vi "Auto 11.vi"(8 "Error In":errorcluster, 11 "Forward?":bool) -> (0 "Error Out":errorcluster)   [LabVIEW 2014]
uses:
  <vilib>/Rock Robotics/Network Tables/SD Read Number.vi
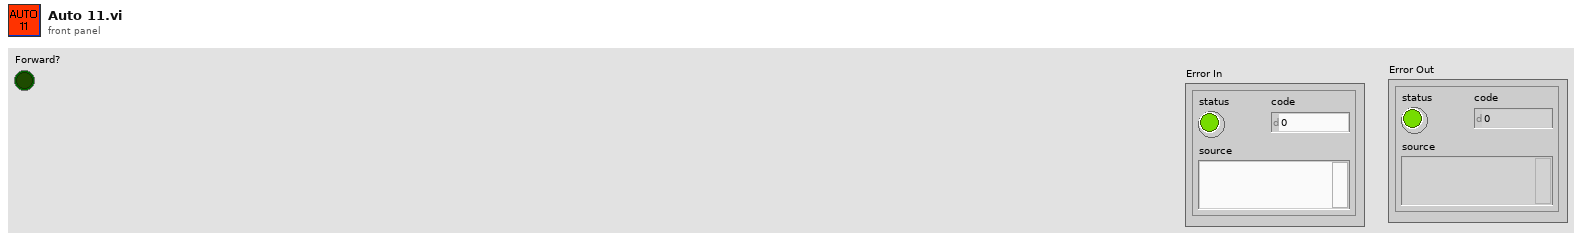
[diagram p1: front panel]
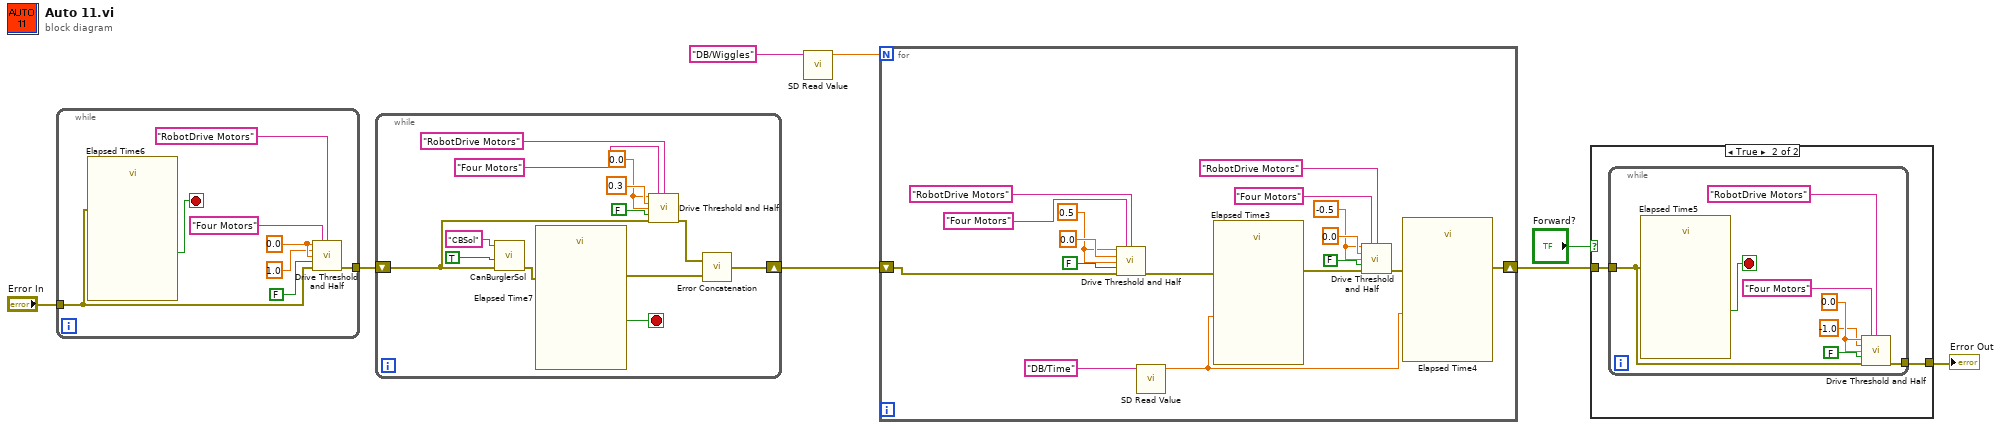
[diagram p0: block diagram]
diagram:
  n1 = while {
    tunnel: [w13] -> w3
    tunnel: "Error In" -> [w10]
    stop <- w11 stop-if-true
    w12 = 0.0 ("Arm Value")
    n2 = call "Elapsed Time6"("error in (no error)"=w10) -> ("Time has Elapsed"=w11:bool)  [unwired: 11 in, 7 out]
    n3 = call "Drive Threshold and Half.vi"("X In"=w12, "Drive refnum name"="Four Motors" ("refnum name"), "Send to DB Name"="RobotDrive Motors" ("Name"), "Y In"=1.0 ("X In"), "R In"=w12, "Speed Toggle"=FALSE ("Grabber Open/Close"), "Error In"=w10) -> ("Error Out"=w13:errorcluster)  [unwired: 8 in]
  }
  n4 = while {
    shift-right: [w17] -> w1
    shift-left: w3 -> [w20]
    stop <- w26 stop-if-true
    w24 = 0.0 ("Arm Value")
    n5 = call "CanBurglerSol.vi"("Error In"=w20, "Grabber Open/Close"=TRUE, "refnum name"="CBSol") -> ("Error Out"=w27:errorcluster)  [unwired: 8 in]
    n6 = call "Elapsed Time7"("error in (no error)"=w27) -> ("Time has Elapsed"=w26:bool, "error out"=w18:errorcluster)  [unwired: 11 in, 6 out]
    n7 = call "Drive Threshold and Half.vi"("X In"=w24, "Drive refnum name"="Four Motors" ("refnum name"), "Send to DB Name"="RobotDrive Motors" ("Name"), "Y In"=0.3 ("X In"), "R In"=w24, "Speed Toggle"=FALSE ("Grabber Open/Close"), "Error In"=w20) -> ("Error Out"=w19:errorcluster)  [unwired: 8 in]
    n8 = call "Error Concatenation.vi"("error in (no error) 2"=w18, "error in (no error)"=w19) -> ("error out"=w17:errorcluster)
  }
  n9 = call-poly <vilib>:"SD Read Value.vi"("Name"="DB/Wiggles") -> ("Numeric"=w4:dbl)  [unwired: 8 in, 2 out]
  n10 = for {
    N: w4 -> [_]
    shift-right: [w34] -> w7
    shift-left: w1 -> [w36]
    w31 = -0.5 ("Arm Value")
    w32 = 0.5 ("Arm Value")
    n11 = call "Drive Threshold and Half.vi"("X In"=w32, "Drive refnum name"="Four Motors" ("refnum name"), "Send to DB Name"="RobotDrive Motors" ("Name"), "Y In"=0.0 ("X In"), "R In"=w32, "Speed Toggle"=FALSE ("Grabber Open/Close"), "Error In"=w36) -> ("Error Out"=w42:errorcluster)  [unwired: 8 in]
    n12 = call-poly <vilib>:"SD Read Value.vi"("Name"="DB/Time") -> ("Numeric"=w30:dbl)  [unwired: 8 in, 2 out]
    n13 = call "Elapsed Time3"("Time Target (s)"=w30, "error in (no error)"=w42) -> ("error out"=w35:errorcluster)  [unwired: 10 in, 7 out]
    n14 = call "Drive Threshold and Half.vi"("X In"=w31, "Drive refnum name"="Four Motors" ("refnum name"), "Send to DB Name"="RobotDrive Motors" ("Name"), "Y In"=0.0 ("X In"), "R In"=w31, "Speed Toggle"=FALSE ("Grabber Open/Close"), "Error In"=w35) -> ("Error Out"=w41:errorcluster)  [unwired: 8 in]
    n15 = call "Elapsed Time4"("Time Target (s)"=w30, "error in (no error)"=w41) -> ("error out"=w34:errorcluster)  [unwired: 10 in, 7 out]
  }
  n16 = case shown="True" "Forward?" {
    tunnel: w7 -> [w47 w49]
    tunnel: [w47 w48] -> w6
    frame False {
    }
    frame True {
      n17 = while {
        tunnel: [w54] -> w48
        tunnel: w49 -> [w51]
        stop <- w52 stop-if-true
        w53 = 0.0 ("Arm Value")
        n18 = call "Elapsed Time5"("error in (no error)"=w51) -> ("Time has Elapsed"=w52:bool)  [unwired: 11 in, 7 out]
        n19 = call "Drive Threshold and Half.vi"("X In"=w53, "Drive refnum name"="Four Motors" ("refnum name"), "Send to DB Name"="RobotDrive Motors" ("Name"), "Y In"=-1.0 ("X In"), "R In"=w53, "Speed Toggle"=FALSE ("Grabber Open/Close"), "Error In"=w51) -> ("Error Out"=w54:errorcluster)  [unwired: 8 in]
      }
    }
  }
  "Error Out" <- w6
